vi "GOOP_DrawWirePreview_ZoomImage.vi"(1 "image data 2":T1, 2 "Zoom":i32=2) -> (0 "image data":T1)   [LabVIEW 2012]
uses:
  <vilib>/picture/picture.llb/imagedata.ctl
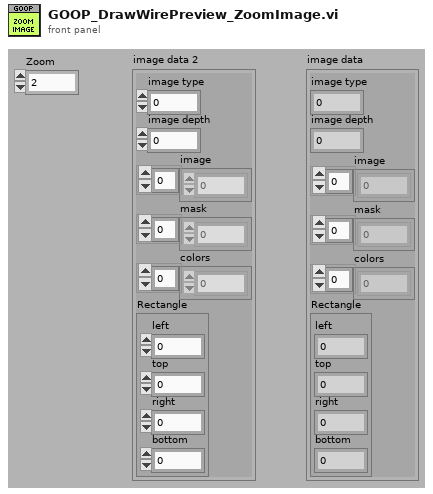
[diagram p1: front panel]
types:
  T1 = typedef "imagedata.ctl" = cluster{"image type":i32, "image depth":i32, "image":u8[], "mask":u8[], "colors":u32[], "Rectangle":cluster{"left":i16, "top":i16, "right":i16, "bottom":i16}}
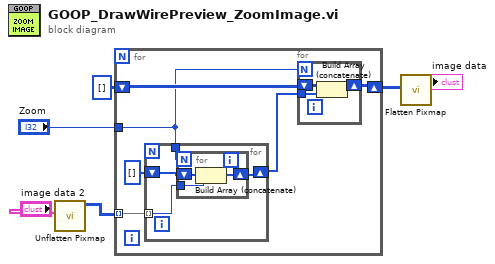
[diagram p0: block diagram]
diagram:
  n1 = call <vilib>:"Unflatten Pixmap.vi"("image data"="image data 2") -> ("24-bit pixmap"=w1:u32[][])  [unwired: 4 in, 6 out]
  n2 = for {
    tunnel: w1 -> [w12] mode=indexing
    tunnel: "Zoom" -> [w7]
    shift-right: [w8] -> w5
    shift-left: u32[][] [] -> [w9]
    n3 = for {
      tunnel: w12 -> [w19] mode=indexing
      shift-right: [w17] -> w10
      shift-left: u8[] [] -> [w18]
      tunnel: w7 -> [w16]
      n4 = for {
        N: w16 -> [_]
        tunnel: w19 -> [w22]
        shift-right: [w20] -> w17
        shift-left: w18 -> [w21]
        n5 = Build Array (concatenate)(w21, w22) -> (w20:u32[])
      }
    }
    n6 = for {
      N: w7 -> [_]
      tunnel: w10 -> [w15]
      shift-right: [w14] -> w8
      shift-left: w9 -> [w13]
      n7 = Build Array (concatenate)(w13, w15) -> (w14:u32[][])
    }
  }
  n8 = call <vilib>:"Flatten Pixmap.vi"("24-bit pixmap"=w5) -> ("image data"=→"image data":T1)  [unwired: 10 in]
